vi "ParseValue.vi"(8 "error in (no error)":errorcluster, 10 "Index In":i32, 11 "JSON String":string) -> (0 "error out":errorcluster, 2 "Index Out":i32, 3 "JSON Tree":variant)   [LabVIEW 2013, in "i3-json.lvlib"]
doc: "Use this template to build a VI to use as a subVI."
uses:
  i3-json.lvlib
  JSON Types/JSON Type.ctl
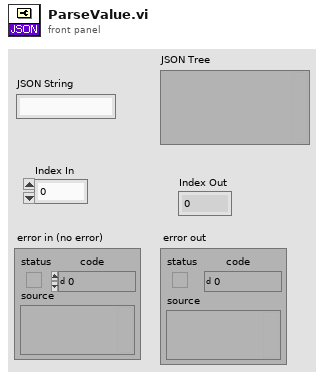
[diagram p1: front panel]
types:
  T1 = typedef "i3-json.lvlib/JSON Type.ctl" = enum8{"JSON Compatible", "JSON Array", "JSON Object", "JSON Null", "Double", "String", "Boolean", "Unknown", "Data JSON string"}
  T2 = typedef "i3-json.lvlib/Token.ctl" = enum16{"NONE", "CURLY_OPEN", "CURLY_CLOSE", "SQUARED_OPEN", "SQUARED_CLOSE", "COLON", "COMMA", "STRING", "NUMBER", "TRUE", "FALSE", "NULL"}
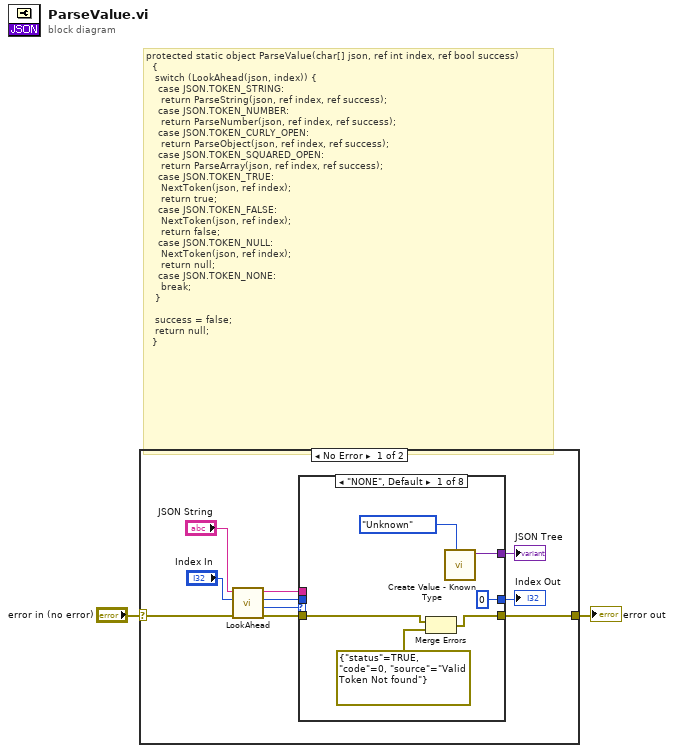
[diagram p0: block diagram]
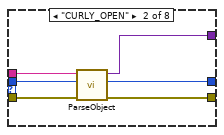
[diagram p2: hidden frame]
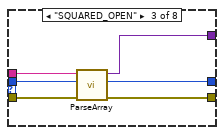
[diagram p3: hidden frame]
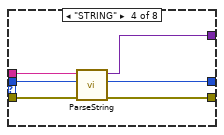
[diagram p4: hidden frame]
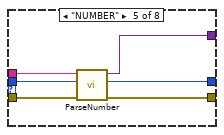
[diagram p5: hidden frame]
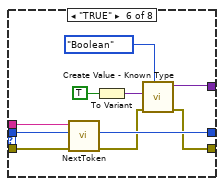
[diagram p6: hidden frame]
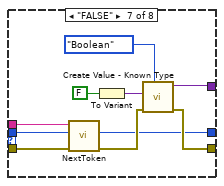
[diagram p7: hidden frame]
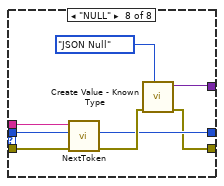
[diagram p8: hidden frame]
diagram:
  # "protected static object ParseValue(char[] json, ref int index, ref bool success)\n\t\t{\n\t\t\tswitch (LookAhead(json, index)) {\n\t\t\t\tcase JSON.TOKEN_STRING:\n\t\t\t\t\treturn ParseString(json, ref index, ref success);\n\t\t\t\tcase JSON.TOKEN_NUMBER:\n\t\t\t\t\treturn ParseNumber(json, ref index, ref success);\n\t\t\t\tcase JSON.TOKEN_CURLY_OPEN:\n\t\t\t\t\treturn ParseObject(json, ref index, ref success);\n\t\t\t\tcase JSON.TOKEN_SQUARED_OPEN:\n\t\t\t\t\treturn ParseArray(json, ref index, ref success);\n\t\t\t\tcase JSON.TOKEN_TRUE:\n\t\t\t\t\tNextToken(json, ref index);\n\t\t\t\t\treturn true;\n\t\t\t\tcase JSON.TOKEN_FALSE:\n\t\t\t\t\tNextToken(json, ref index);\n\t\t\t\t\treturn false;\n\t\t\t\tcase JSON.TOKEN_NULL:\n\t\t\t\t\tNextToken(json, ref index);\n\t\t\t\t\treturn null;\n\t\t\t\tcase JSON.TOKEN_NONE:\n\t\t\t\t\tbreak;\n\t\t\t}\n\n\t\t\tsuccess = false;\n\t\t\treturn null;\n\t\t}"
  n1 = case shown="No Error" "error in (no error)" {
    selector: "error in (no error)" -> [w10 w71]
    tunnel: [w8 w71] -> w1
    frame No Error {
      n2 = call "LookAhead.vi"("error in (no error)"=w10, "Index"="Index In", "JSON String"="JSON String") -> ("error out"=w9:errorcluster, "TOKEN"=w6:T2, "Index Passthrough"=w4:i32, "JSON String Passthrough"=w5:string)  [unwired: 4 in]
      n3 = case shown="\"NONE\", Default" w6 {
        tunnel: w9 -> [w14 w22 w28 w34 w40 w49 w55 w66]
        tunnel: [w15 w21 w27 w33 w39 w48 w57 w64] -> w8
        tunnel: [w17 w19 w25 w31 w37 w47 w58 w63] -> w7
        tunnel: w5 -> [_ w23 w30 w36 w42 w52 w53 w68]
        tunnel: w4 -> [_ w24 w29 w35 w41 w51 w54 w67]
        tunnel: [0 ("Index Out") w20 w26 w32 w38 w50 w56 w65] -> w3
        frame "NONE", Default {
          n4 = Merge Errors(w14, errorcluster {"status"=TRUE, "code"=0, "source"="Valid Token Not found"} ("error out")) -> (w15:errorcluster)
          n5 = call "Create Value - Known Type.vi"("JSON Type"=JSON_Type."Unknown") -> ("JSON Tree"=w17:variant)  [unwired: 9 in, 1 out]
        }
        frame "CURLY_OPEN" {
          n6 = call "ParseObject.vi"("error in (no error)"=w22, "Index In"=w24, "JSON String"=w23) -> ("error out"=w21:errorcluster, "Index Out"=w20:i32, "JSON Tree"=w19:variant)  [unwired: 6 in]
        }
        frame "SQUARED_OPEN" {
          n7 = call "ParseArray.vi"("error in (no error)"=w28, "Index In"=w29, "JSON String"=w30) -> ("error out"=w27:errorcluster, "Index Out"=w26:i32, "JSON Tree"=w25:variant)  [unwired: 6 in]
        }
        frame "STRING" {
          n8 = call "ParseString.vi"("error in (no error)"=w34, "Index In"=w35, "JSON String"=w36) -> ("error out"=w33:errorcluster, "Index Out"=w32:i32, "JSON Tree"=w31:variant)  [unwired: 5 in, 1 out]
        }
        frame "NUMBER" {
          n9 = call "ParseNumber.vi"("error in (no error)"=w40, "Index In"=w41, "JSON String"=w42) -> ("error out"=w39:errorcluster, "Index Out"=w38:i32, "JSON Tree"=w37:variant)  [unwired: 6 in]
        }
        frame "TRUE" {
          n10 = call "NextToken.vi"("error in (no error)"=w49, "Index In"=w51, "JSON String"=w52) -> ("error out"=w46:errorcluster, "Index Out"=w50:i32)  [unwired: 4 in, 2 out]
          n11 = To Variant(anything=TRUE) -> (Variant=w43:variant)
          n12 = call "Create Value - Known Type.vi"("JSON Type"=JSON_Type."Boolean", "error in (no error)"=w46, "Value"=w43) -> ("error out"=w48:errorcluster, "JSON Tree"=w47:variant)  [unwired: 7 in]
        }
        frame "FALSE" {
          n13 = call "NextToken.vi"("error in (no error)"=w55, "Index In"=w54, "JSON String"=w53) -> ("error out"=w62:errorcluster, "Index Out"=w56:i32)  [unwired: 4 in, 2 out]
          n14 = To Variant(anything=FALSE) -> (Variant=w59:variant)
          n15 = call "Create Value - Known Type.vi"("JSON Type"=JSON_Type."Boolean", "error in (no error)"=w62, "Value"=w59) -> ("error out"=w57:errorcluster, "JSON Tree"=w58:variant)  [unwired: 7 in]
        }
        frame "NULL" {
          n16 = call "NextToken.vi"("error in (no error)"=w66, "Index In"=w67, "JSON String"=w68) -> ("error out"=w70:errorcluster, "Index Out"=w65:i32)  [unwired: 4 in, 2 out]
          n17 = call "Create Value - Known Type.vi"("JSON Type"=JSON_Type."JSON Null", "error in (no error)"=w70) -> ("error out"=w64:errorcluster, "JSON Tree"=w63:variant)  [unwired: 8 in]
        }
      }
      "JSON Tree" <- w7
      "Index Out" <- w3
    }
    frame Error {
    }
  }
  "error out" <- w1
